vi "UpdateGridPoint.vi"(0 "object in":refnum<class "Map.lvclass">, 2 "Coordinates":T2, 3 "State":T1, 5 "error in (no error)":errorcluster) -> (14 "object out":refnum<class "Map.lvclass">, 16 "Grid":u32[][](array[colorbox]), 19 "error out":errorcluster)   [LabVIEW 2015, in "Map.lvclass"]
doc: "Changes the state of one grid point on the map."
uses:
  Map.lvclass
  TypDefs/Coordinates.ctl
  TypDefs/GridState.ctl
  Map.lvclass/Map.ctl
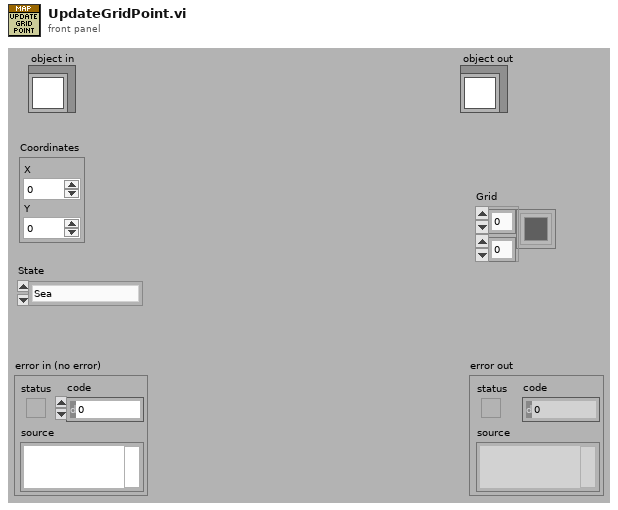
[diagram p1: front panel]
types:
  T1 = typedef "GridState.ctl" = enum16{"Sea", "Ship", "Hit", "Miss"}
  T2 = typedef "Coordinates.ctl" = cluster{"X":i32, "Y":i32}
  T3 = cluster{"Sea":u32, "Ship":u32, "Hit":u32, "Miss":u32}
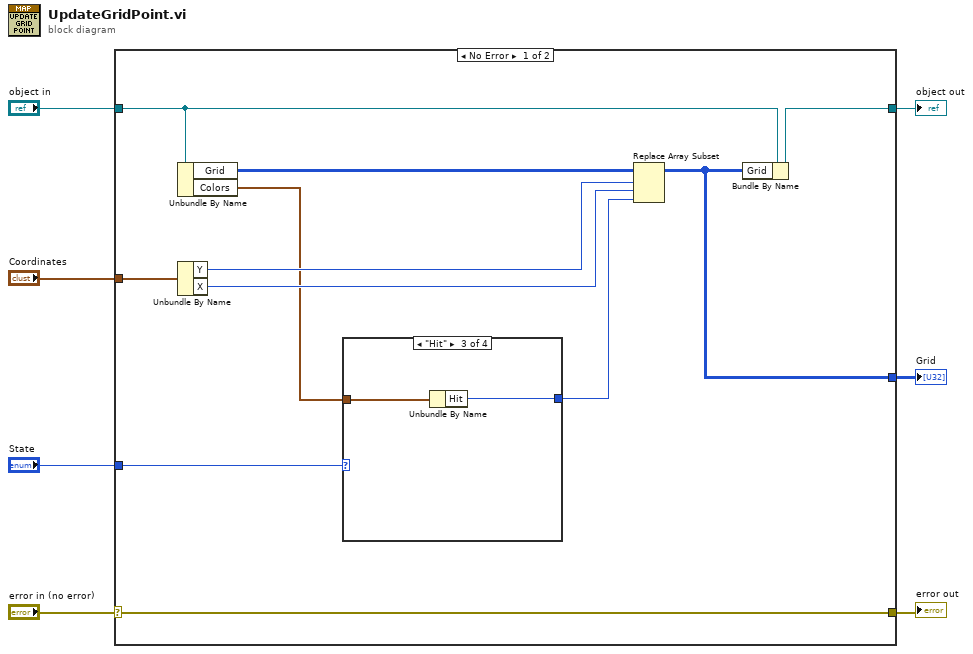
[diagram p0: block diagram]
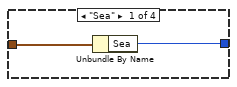
[diagram p2: hidden frame]
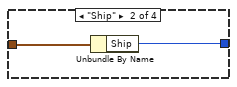
[diagram p3: hidden frame]
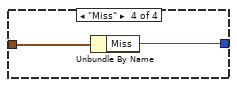
[diagram p4: hidden frame]
diagram:
  n1 = case shown="No Error" "error in (no error)" {
    selector: "error in (no error)" -> [w18 w28]
    tunnel: [w18 w28] -> w6
    tunnel: [w16 w27] -> w4
    tunnel: "object in" -> [w17 w27]
    tunnel: "Coordinates" -> [w14 _]
    tunnel: [w9 _] -> w2
    tunnel: "State" -> [w8 _]
    frame No Error {
      n2 = Unbundle By Name(w17) -> ("Grid"=w15:u32[][], "Colors"=w11:T3)
      n3 = Unbundle By Name(w14) -> ("Y"=w13:i32, "X"=w12:i32)
      n4 = case shown="\"Hit\"" w8 {
        tunnel: w11 -> [w20 w22 w24 w26]
        tunnel: [w19 w21 w23 w25] -> w10
        frame "Sea" {
          n5 = Unbundle By Name(w20) -> ("Sea"=w19:u32)
        }
        frame "Ship" {
          n6 = Unbundle By Name(w22) -> ("Ship"=w21:u32)
        }
        frame "Hit" {
          n7 = Unbundle By Name(w24) -> ("Hit"=w23:u32)
        }
        frame "Miss" {
          n8 = Unbundle By Name(w26) -> ("Miss"=w25:u32)
        }
      }
      n9 = Replace Array Subset(array=w15, new element=w10, index (row)=w13, index (col)=w12) -> (w9:u32[][])
      n10 = Bundle By Name(cluster=w17, "Grid"=w9) -> (w16:refnum<class "Map.lvclass">)
    }
    frame Error {
    }
  }
  "error out" <- w6
  "object out" <- w4
  "Grid" <- w2
